vi "Final.vi"() -> ()   [LabVIEW 2019]
doc: "The myRIO Project template acquires acceleration data from the onboard accelerometer and displays the changes of acceleration values in a waveform chart."
uses:
  <vilib>/myRIO/Instrument Drivers/Onboard IO/I2C/typedefs/I2C User Configuration.ctl
  <vilib>/myRIO/Instrument Drivers/Onboard IO/I2C/typedefs/I2C Transfer Rate.ctl
  <vilib>/Platform/TimedLoop/XDataNode/timing_clust.ctl
  <vilib>/Platform/TimedLoop/XDataNode/nitl_modes.ctl
  <vilib>/Platform/TimedLoop/XDataNode/wakeup.ctl
  <vilib>/myRIO/Instrument Drivers/Onboard Devices/Accelerometer/typedefs/Accelerometer Reference.ctl
  <vilib>/myRIO/Common/Instrument Driver Framework/Utilities/typedefs/myRIO Generic Hardware Reference.ctl
  <vilib>/myRIO/Common/Instrument Driver Framework/Utilities/typedefs/Hardware Version Enum.ctl
  <vilib>/myRIO/Common/Instrument Driver Framework/Utilities/typedefs/myRIO v1.0 Reference.ctl
  <vilib>/myRIO/Common/Instrument Driver Framework/Utilities/typedefs/Generic FPGA Reference.ctl
  <vilib>/myRIO/Common/Instrument Driver Framework/myRIO v1.0/Accelerometer/typedefs/Accelerometer Channels List.ctl
  <vilib>/myRIO/Common/Instrument Driver Framework/myRIO v1.0/Accelerometer/typedefs/Accelerometer Channels Enum.ctl
  <vilib>/userDefined/High Color/nirio_resource_hc.ctl
  <vilib>/myRIO/Instrument Drivers/Onboard IO/PWM/typedefs/PWM Reference.ctl
  <vilib>/myRIO/Common/Instrument Driver Framework/myRIO v1.0/PWM/typedefs/PWM Channels Enum.ctl
  <vilib>/myRIO/Instrument Drivers/Onboard IO/PWM/typedefs/PWM Configuration.ctl
  <vilib>/myRIO/Instrument Drivers/Onboard IO/DIO/typedefs/DIO Reference.ctl
  <vilib>/myRIO/Common/Instrument Driver Framework/myRIO v1.0/DIO/typedefs/DIO Channels List.ctl
  <vilib>/myRIO/Common/Instrument Driver Framework/myRIO v1.0/DIO/typedefs/DIO Channels Enum.ctl
  <vilib>/myRIO/Common/Instrument Driver Framework/Utilities/vis/Is FPGA Ref Available.vi
  <vilib>/myRIO/Common/Instrument Driver Framework/myRIO v1.0/Accelerometer/vis/myRIO v1.1 Open Accelerometer.vi
  <vilib>/myRIO/Common/Instrument Driver Framework/myRIO v1.0/PWM/vis/myRIO v1.1 Open PWM.vi
  <vilib>/myRIO/Instrument Drivers/Onboard IO/PWM/vis/Set Duty Cycle and Frequency.vi
  <vilib>/myRIO/Common/Instrument Driver Framework/myRIO v1.0/DIO/vis/myRIO v1.1 Open DIO.vi
  <vilib>/myRIO/Common/Instrument Driver Framework/myRIO v1.0/I2C/vis/myRIO v1.1 Open I2C.vi
  <vilib>/myRIO/Common/Instrument Driver Framework/Utilities/vis/Validate Channels.vi
  <vilib>/myRIO/Common/Instrument Driver Framework/myRIO v1.0/Accelerometer/vis/myRIO v1.0 Reserve Accelerometer.vi
  <vilib>/myRIO/Common/Instrument Driver Framework/myRIO v1.0/PWM/vis/myRIO v1.0 Reserve PWM.vi
  <vilib>/myRIO/Common/Instrument Driver Framework/myRIO v1.0/DIO/vis/myRIO v1.0 Reserve DIO.vi
  <vilib>/myRIO/Common/Instrument Driver Framework/myRIO v1.0/UART/vis/myRIO v1.0 Close UART.vi
  <vilib>/myRIO/Common/Instrument Driver Framework/myRIO v1.0/I2C/vis/myRIO v1.0 Reserve I2C.vi
  <vilib>/myRIO/Common/Instrument Driver Framework/myRIO v1.0/Resource Manager/vis/myRIO v1.0 Reserve Channel List.vi
  <vilib>/myRIO/Common/Instrument Driver Framework/myRIO v1.0/Accelerometer/vis/myRIO v1.0 Build MUX Configuration Accelerometer.vi
  <vilib>/myRIO/Common/Instrument Driver Framework/myRIO v1.0/PWM/vis/myRIO v1.0 Build MUX Configuration PWM.vi
  <vilib>/myRIO/Common/Instrument Driver Framework/myRIO v1.0/DIO/vis/myRIO v1.0 Build MUX Configuration DIO.vi
  <vilib>/myRIO/Common/Instrument Driver Framework/myRIO v1.0/I2C/vis/myRIO v1.0 Build MUX Configuration I2C.vi
  <vilib>/myRIO/Common/Instrument Driver Framework/myRIO v1.0/Resource Manager/vis/myRIO v1.0 Reserve Channel.vi
  <vilib>/myRIO/Common/Instrument Driver Framework/myRIO v1.0/Resource Manager/vis/myRIO v1.0 Unreserve Channel.vi
  <vilib>/myRIO/Common/Instrument Driver Framework/myRIO v1.0/Resource Manager/vis/myRIO v1.0 Create Configuration List.vi
  <vilib>/myRIO/Common/Instrument Driver Framework/myRIO v1.0/Resource Manager/vis/myRIO v1.0 Build Mutex Name.vi
  <vilib>/Utility/VariantDataType/GetNumericInfo.vi
  <vilib>/Utility/error.llb/Error Cluster From Error Code.vi
  <vilib>/myRIO/Common/Instrument Driver Framework/myRIO v1.0/myRIO v1.1 Open.vi
  <vilib>/myRIO/Common/Instrument Driver Framework/Utilities/vis/IO Manager.vi
  <vilib>/myRIO/Common/Instrument Driver Framework/Utilities/vis/Configuration Manager.vi
  <vilib>/myRIO/Common/Instrument Driver Framework/myRIO v1.0/Resource Manager/vis/myRIO v1.0 Configure IO.vi
  <vilib>/myRIO/Common/Instrument Driver Framework/myRIO v1.0/myRIO v1.0 Close.vi
  <vilib>/myRIO/Common/Instrument Driver Framework/myRIO v1.0/I2C/vis/myRIO v1.0 Configure I2C.vi
  <vilib>/myRIO/Common/Instrument Driver Framework/myRIO v1.0/I2C/vis/myRIO v1.0 Write I2C.vi
  <vilib>/myRIO/Common/Instrument Driver Framework/myRIO v1.0/Accelerometer/vis/myRIO v1.0 Get Scaling Constant Accelerometer.vi
  <vilib>/myRIO/Common/Instrument Driver Framework/myRIO v1.0/Accelerometer/vis/myRIO v1.0 Read Accelerometer.vi
  <vilib>/myRIO/Common/Instrument Driver Framework/myRIO v1.0/DIO/vis/myRIO v1.0 Read DIO.vi
  <vilib>/myRIO/Common/Instrument Driver Framework/myRIO v1.0/DIO/vis/myRIO v1.0 Write DIO.vi
  <vilib>/myRIO/Common/Instrument Driver Framework/myRIO v1.0/I2C/vis/myRIO v1.0 Read I2C.vi
  <vilib>/myRIO/Common/Instrument Driver Framework/myRIO v1.0/PWM/vis/myRIO v1.0 Write PWM.vi
  <vilib>/myRIO/Common/Instrument Driver Framework/Utilities/vis/FPGA Ref Manager.vi
  <vilib>/myRIO/Common/Instrument Driver Framework/myRIO v1.0/myRIO v1.0 Reset FPGA.vi
  <vilib>/myRIO/Common/Instrument Driver Framework/myRIO v1.0/IRQ/vis/myRIO v1.0 IRQ Info FGV.vi
  <vilib>/myRIO/Common/Instrument Driver Framework/myRIO v1.0/IRQ/vis/myRIO v1.0 Timer IRQ Info FGV.vi
  <vilib>/myRIO/Common/Instrument Driver Framework/myRIO v1.0/IRQ/vis/myRIO v1.0 ISR Agent.vi
  <vilib>/myRIO/Instrument Drivers/Utilities/vis/Reset Index.vi
  <vilib>/myRIO/Common/Instrument Driver Framework/myRIO v1.0/Resource Manager/vis/myRIO v1.0 Block Write Resource Manager.vi
  <vilib>/Platform/TimedLoop/XDataNode/XDataNode.xnode
  <vilib>/myRIO/Express VI/Onboard Devices/Accelerometer/Accelerometer Express VI.xnode
  <vilib>/myRIO/Instrument Drivers/Onboard Devices/Accelerometer/vis/myRIO Accelerometer Open.xnode
  <vilib>/myRIO/Express VI/Onboard IO/PWM/PWM Express VI.xnode
  <vilib>/myRIO/Instrument Drivers/Onboard IO/PWM/vis/myRIO PWM Open.xnode
  <vilib>/myRIO/Express VI/Onboard IO/DO/DO Express VI.xnode
  <vilib>/myRIO/Instrument Drivers/Onboard IO/DIO/vis/myRIO DIO Open.xnode
  <vilib>/myRIO/Instrument Drivers/Onboard IO/I2C/I2C.lvlib
  <vilib>/myRIO/Instrument Drivers/Onboard IO/DIO/DIO.lvlib
  <vilib>/myRIO/Instrument Drivers/Utilities/Utilities.lvlib
  <vilib>/myRIO/Instrument Drivers/Onboard IO/PWM/PWM.lvlib
  <vilib>/addons/control/pid/NI_PID_autopid.lvlib
  <vilib>/Platform/TimedLoop/XDataNode/XDNodeRunTimeDep.lvlib
  <vilib>/myRIO/Instrument Drivers/Onboard Devices/Accelerometer/Accelerometer.lvlib
panel:
  out "output":dbl(graph) caption="출력"
  in  "[ESC]":bool
  out "X rate":i16
  out "Y rate":i16
  out "Z rate":i16
  out "DATA":u8[](array[numeric]) format="%02x"
  out "Angular rate [LSB/sec]":cluster{i16, i16, i16}(graph)
  in  "break":bool
  in  "dead":dbl format="%#_13g"
  out "abs(x)":dbl
  out "x*y":dbl
  out "숫자형 컨트롤 2":dbl
  in  "setpoint 2":dbl caption="셋포인트" format="%.2f"
  out "웨이브폼 차트 2":dbl(graph)
  in  "PID gains 3":T1={"proportional gain (Kc)"=1.0, "integral time (Ti, min)"=0.01, "derivative time (Td, min)"=0.0} {"proportional gain (Kc)" step=1.0; "integral time (Ti, min)" step=1.0; "derivative time (Td, min)" step=1.0}
  out "PID gains out":T1={"proportional gain (Kc)"=1.0, "integral time (Ti, min)"=0.01, "derivative time (Td, min)"=0.0} caption="PID 게인 출력" {"derivative time (Td, min)" format="%.3f"; "integral time (Ti, min)" format="%.3f"; "proportional gain (Kc)" format="%.3f"}
  in  "autotune? (F)":bool caption="자동튜닝? (거짓)"
  in  "autotuning parameters":T2={"controller type"=1, "relay cycles"=3, "relay amplitude"=1.0, "control specification"=2, "PV noise level"=0.1} caption="자동튜닝 파라미터" {"PV noise level" format="%.2f"; "control specification" items=["보통", "빠르게", "느리게"]; "relay amplitude" format="%.2f"; "controller type" items=["PID", "PI", "P"]}
  out "tuning completed?":bool caption="튜닝 완료?"
  out "dt out (s)":dbl caption="dt 출력 (초)" format="%.3f"
  in  "reinitialize? (F)":bool caption="다시 초기화? (거짓)"
  out "숫자형 컨트롤":dbl
  # "Overview: The myRIO Project template acquires acceleration data from the onboard accelerometer and displays the changes of acceleration values in a waveform chart.\nInstructions:\n1. Check the myRIO target IP address in the project and make sure the target IP address is correct. \n2. Run this VI."
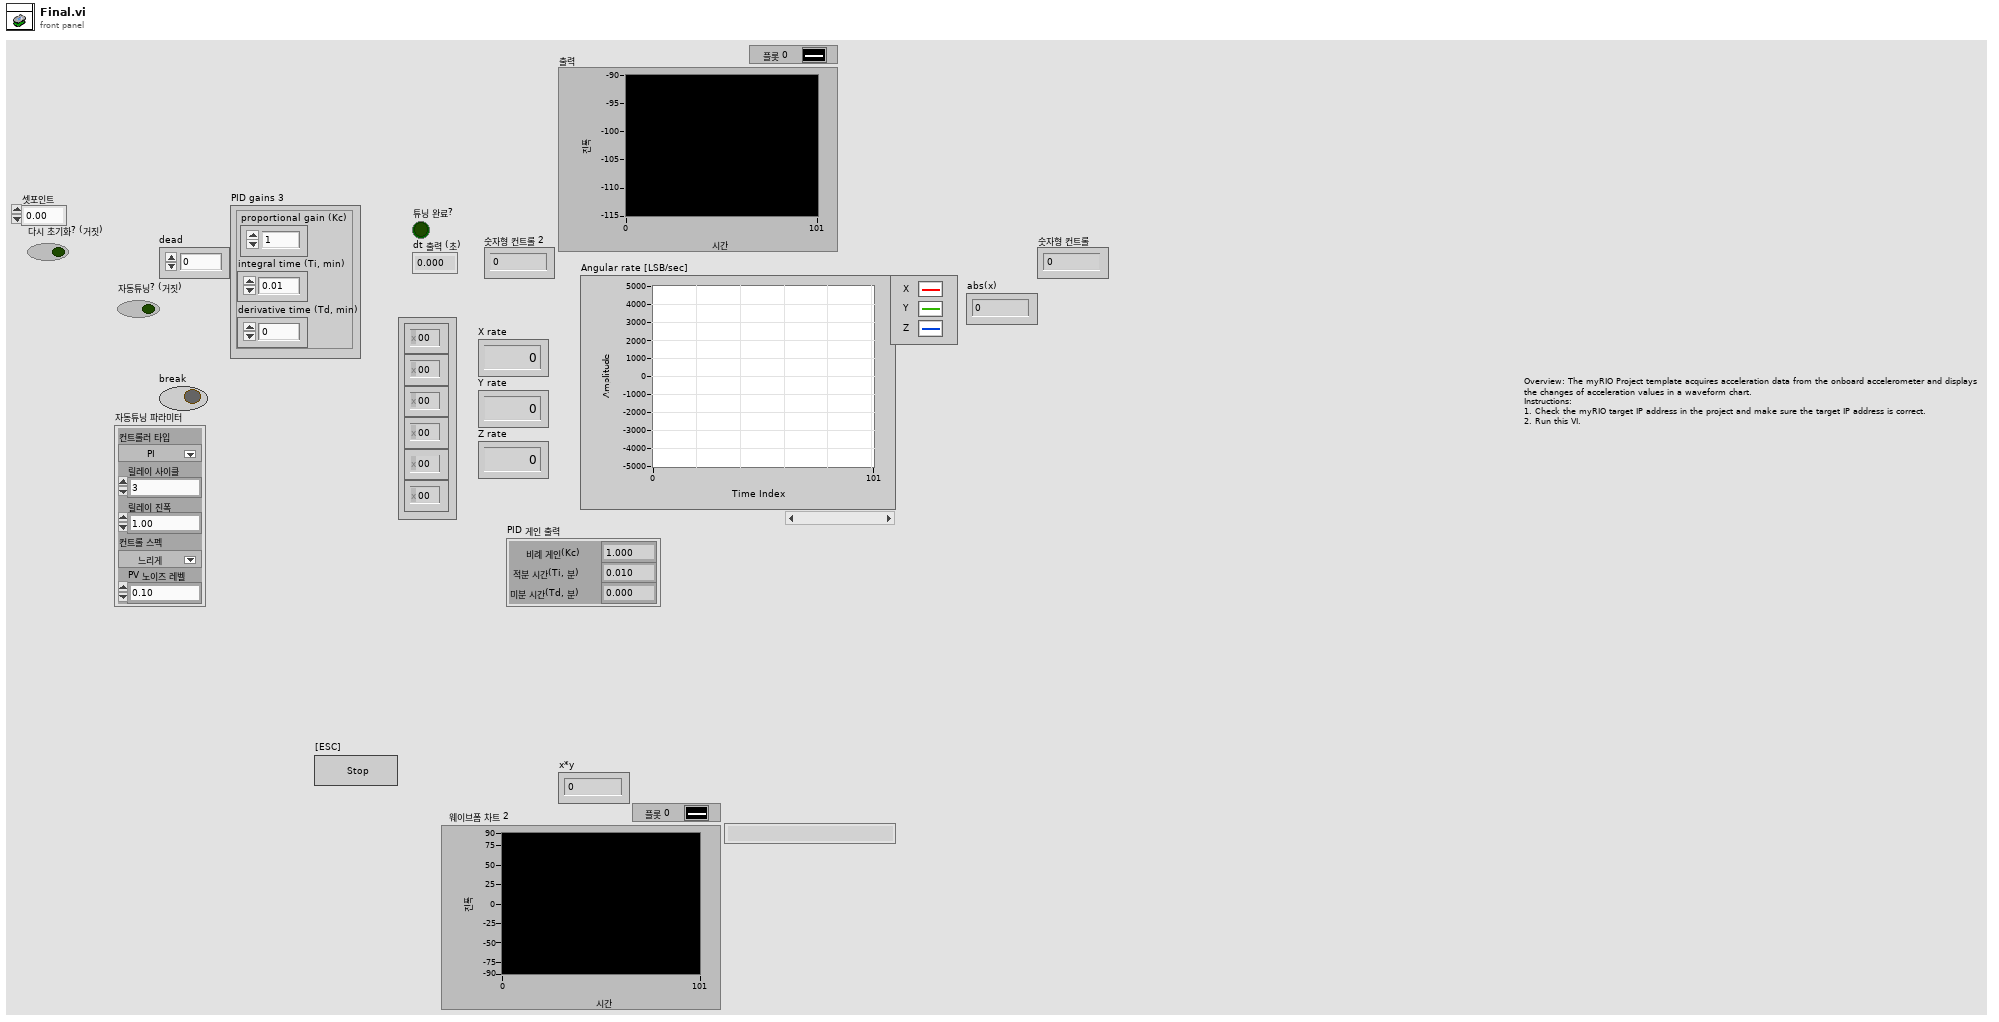
[diagram p1: front panel]
types:
  T1 = cluster{"proportional gain (Kc)":dbl, "integral time (Ti, min)":dbl, "derivative time (Td, min)":dbl}
  T2 = cluster{"controller type":u16, "relay cycles":i32, "relay amplitude":dbl, "control specification":u16, "PV noise level":dbl}
  T3 = typedef "I2C.lvlib/I2C User Configuration.ctl" = cluster{"I2C Transfer Rate":T4}
  T4 = typedef "I2C.lvlib/I2C Transfer Rate.ctl" = enum16{"Standard mode (100 kbps)", "Fast mode (400 kbps)"}
  T5 = typedef "I2C.lvlib/I2C Reference.ctl" = cluster{"myRIO Reference":T6, "I2C Channels Enum":T10, "I2C Configuration":T11}
  T6 = typedef "myRIO Generic Hardware Reference.ctl" = cluster{"myRIO Model":T7, "myRIO Hardware Reference":T8}
  T7 = typedef "Hardware Version Enum.ctl" = enum16{"Unknown", "myRIO-1900", "myRIO-1950", "roboRIO", "NI ELVIS RIO CM", "ELVIS III"}
  T8 = typedef "myRIO v1.0 Reference.ctl" = cluster{"Generic FPGA Reference":T9, "Allow multiple opens":bool}
  T9 = typedef "Generic FPGA Reference.ctl" = refnum<k20>
  T10 = typedef "I2C Channels Enum.ctl" = enum16{"Not Connected", "A/I2C", "B/I2C", "I2C/I2C"}
  T11 = typedef "I2C.lvlib/I2C Configuration.ctl" = cluster{"I2C Transfer Rate":T4}
  T12 = typedef "DIO.lvlib/DIO Reference.ctl" = cluster{"myRIO Reference":T6, "DIO Channels List":T13}
  T13 = typedef "DIO Channels List.ctl" = T14[]
  T14 = typedef "DIO Channels Enum.ctl" = enum16{"Not Connected", "C/DIO0", "C/DIO1", "C/DIO2", "C/DIO3", "C/DIO4", "C/DIO5", "C/DIO6", "C/DIO7", "A/DIO0", "A/DIO1", "A/DIO2", "A/DIO3", "A/DIO4", "A/DIO5", "A/DIO6", "A/DIO7", "A/DIO8", "A/DIO9", "A/DIO10", "A/DIO11", "A/DIO12", "A/DIO13", "A/DIO14", "A/DIO15", "A/DIO16", "A/DIO17", "A/DIO18", "A/DIO19", "B/DIO0", "B/DIO1", "B/DIO2", "B/DIO3", "B/DIO4", "B/DIO5", "B/DIO6", "B/DIO7", "B/DIO8", "B/DIO9", "B/DIO10", "B/DIO11", "B/DIO12", "B/DIO13", "B/DIO14", "B/DIO15", "B/DIO16", "B/DIO17", "B/DIO18", "B/DIO19", "LED0", "LED1", "LED2", "LED3", "Button0", "DIO/DIO0", "DIO/DIO1", "DIO/DIO2", "DIO/DIO3", "DIO/DIO4", "DIO/DIO5", "DIO/DIO6", "DIO/DIO7", "DIO/DIO8", "DIO/DIO9", "SPI/CS0", "SPI/CS1", "SPI/CS2", "SPI/CS3", "LED RADIO (Green)", "LED RADIO (Red)", "LED COMM (Green)", "LED COMM (Red)", "LED MODE (Green)", "LED MODE (Red)"}
  T15 = typedef "XDNodeRunTimeDep.lvlib/timing_clust.ctl" = cluster{"Expected End [f-1]":u64, "Actual End [f-1]":u64, "Finished Late? [f-1]":bool, "Expected End [i-1]":u64, "Actual End [i-1]":u64, "Finished Late? [i-1]":bool, "Expected Start [i]":u64, "Actual Start [i]":u64, "Expected Start [f]":u64, "Actual Start [f]":u64, "Source Name":string, "Structure Name":string, "Period":i64, "Deadline":i64, "Offset":i64, "Start":i64, "Priority":i32, "Timeout":i32, "Mode":T16, "Wakeup Reason":T17, "Error":errorcluster, "Source Type":string, "Secondary Source Type":string, "Global End Time":u64, "Global Start Time":u64, "Frame Duration":u64, "Iteration Duration":u64, "Assigned CPU":i32, "I/O Scan Engine Mode":u32}
  T16 = typedef "XDNodeRunTimeDep.lvlib/nitl_modes.ctl" = enum32{"No Change", "Process missed periods, maintain original phase", "Discard missed periods, maintain original phase", "Process missed periods, ignore original phase", "Discard missed periods, ignore original phase"}
  T17 = typedef "XDNodeRunTimeDep.lvlib/wakeup.ctl" = enum32{"Normal", "Aborted", "Asynchronous wakeup", "Timing source error", "Timed loop error", "Timeout"}
  T18 = typedef "Accelerometer.lvlib/Accelerometer Reference.ctl" = cluster{"myRIO Reference":T6, "Accelerometer Channels List":T19, "LSB Weight":dbl}
  T19 = typedef "Accelerometer Channels List.ctl" = T20[]
  T20 = typedef "Accelerometer Channels Enum.ctl" = enum16{"Not Connected", "X-Axis", "Y-Axis", "Z-Axis"}
  T21 = typedef "nirio_resource_hc.ctl" = tag
  T22 = typedef "PWM.lvlib/PWM Reference.ctl" = cluster{"myRIO Reference":T6, "PWM Channels Enum":T23, "PWM Configuration":T24}
  T23 = typedef "PWM Channels Enum.ctl" = enum16{"Not Connected", "C/PWM0", "C/PWM1", "A/PWM0", "A/PWM1", "A/PWM2", "A/PWM3", "A/PWM4", "A/PWM5", "A/PWM6", "A/PWM7", "A/PWM8", "A/PWM9", "A/PWM10", "A/PWM11", "A/PWM12", "A/PWM13", "A/PWM14", "A/PWM15", "A/PWM16", "A/PWM17", "A/PWM18", "A/PWM19", "B/PWM0", "B/PWM1", "B/PWM2", "B/PWM3", "B/PWM4", "B/PWM5", "B/PWM6", "B/PWM7", "B/PWM8", "B/PWM9", "B/PWM10", "B/PWM11", "B/PWM12", "B/PWM13", "B/PWM14", "B/PWM15", "B/PWM16", "B/PWM17", "B/PWM18", "B/PWM19", "PWM/PWM0", "PWM/PWM1", "PWM/PWM2", "PWM/PWM3", "PWM/PWM4", "PWM/PWM5", "PWM/PWM6", "PWM/PWM7", "PWM/PWM8", "PWM/PWM9"}
  T24 = typedef "PWM.lvlib/PWM Configuration.ctl" = cluster{"Frequency":dbl, "Duty Cycle":dbl}
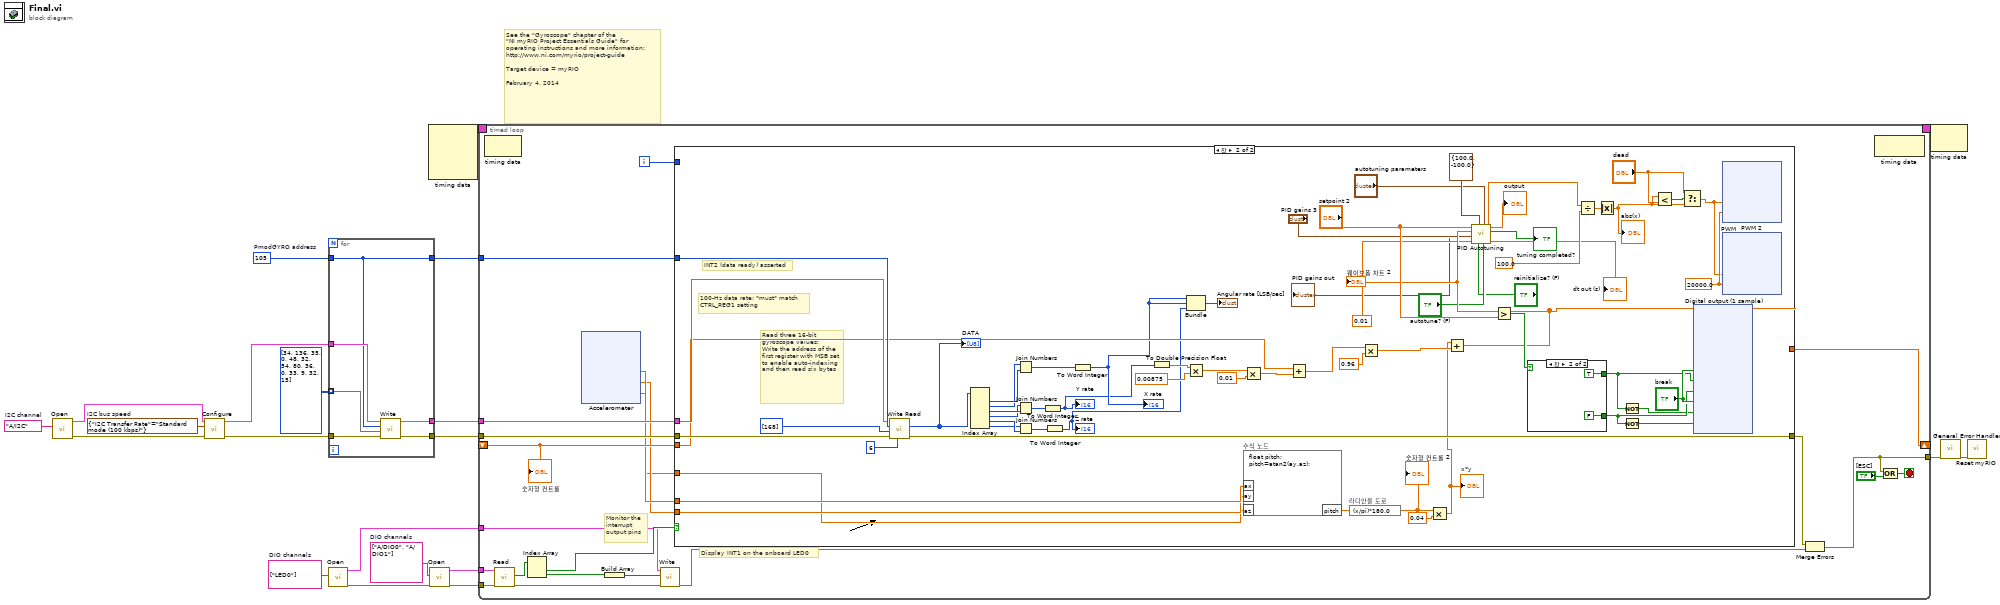
[diagram p0: block diagram]
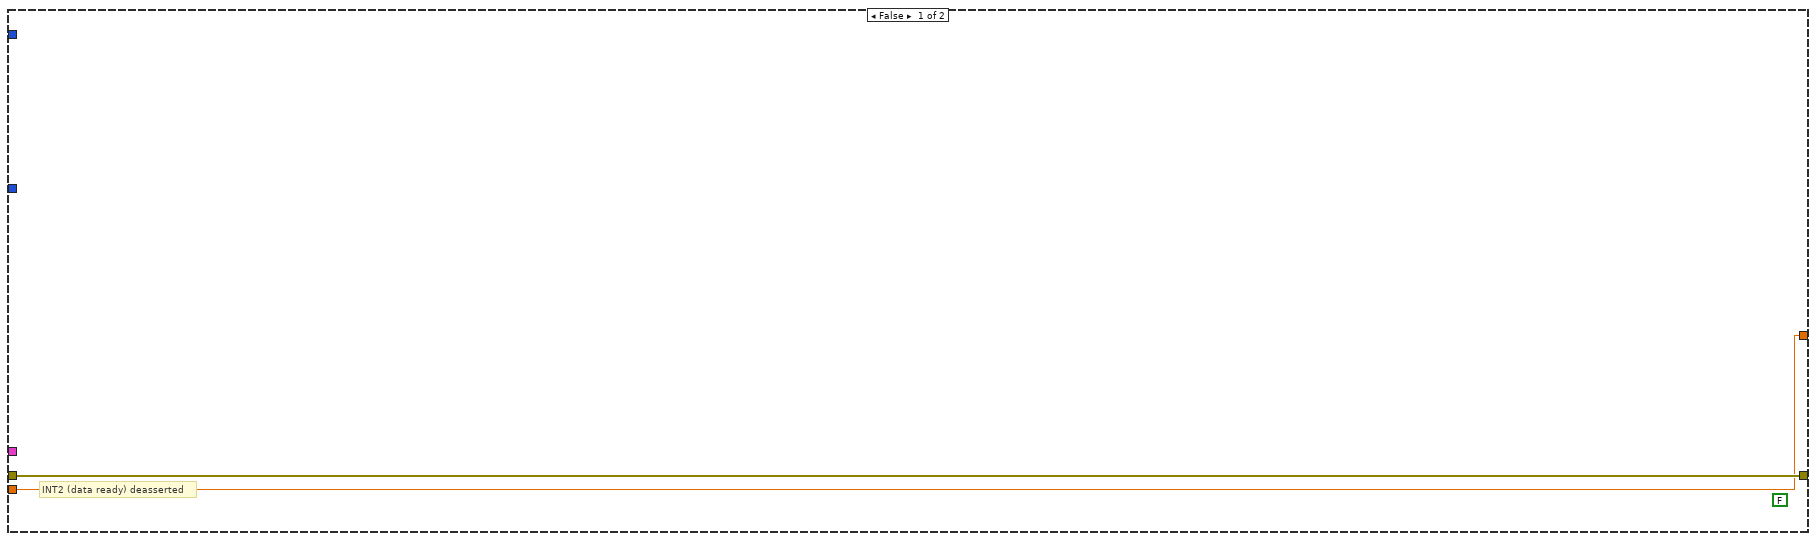
[diagram p2: hidden frame]
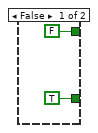
[diagram p3: hidden frame]
diagram:
  w5 = tag[] ["LED0"]  # DIO channels
  w6 = tag[] ["A/DIO0", "A/DIO1"]  # DIO channels
  w18 = T3 {"I2C Transfer Rate"=enum."Standard mode (100 kbps)"}  # I2C bus speed
  w19 = tag "A/I2C"  # I2C channel
  w9 = u8 105  # PmodGYRO address
  # "See the \"Gyroscope\" chapter of the\n\"NI myRIO Project Essentials Guide\" for\noperating instructions and more information: \nhttp://www.ni.com/myrio/project-guide\n\nTarget device = myRIO\n\nFebruary 4, 2014"
  n1 = call <vilib>:"Open.vi"("Channel Name"=w19) -> ("error out"=w16:errorcluster, "I2C Ref Out"=w17:T5)  [unwired: 9 in]
  n2 = call <vilib>:"Configure.vi"("error in (no error)"=w16, "I2C User Configuration"=w18, "I2C Ref In"=w17) -> ("error out"=w10:errorcluster, "I2C Ref Out"=w11:T5)  [unwired: 7 in]
  n3 = for {
    tunnel: [w27] -> w15
    tunnel: [w26] -> w14
    tunnel: [w22] -> w13
    tunnel: u8[][] [[34, 136], [35, 0], [48, 32], [54, 80], [36, 0], [33, 9], [32, 15]] ("Bytes to Write") -> [w25] mode=indexing
    tunnel: w11 -> [w24]
    tunnel: w10 -> [w23]
    tunnel: w9 -> [w22]
    n4 = call <vilib>:"Write.vi"("error in (no error)"=w23, "Bytes to Write"=w25, "Slave Address (7-bit)"=w22, "I2C Ref In"=w24) -> ("error out"=w27:errorcluster, "I2C Ref Out"=w26:T5)  [unwired: 6 in]
  }
  n5 = call <vilib>:"Open.vi"("Channel Names"=w5) -> ("error out"=w3:errorcluster, "DIO Ref Out"=w4:T12)  [unwired: 9 in]
  n6 = node-c288() -> (w21:T15)  [unwired: 4 in]
  n7 = call <vilib>:"Open.vi"("error in (no error)"=w3, "Channel Names"=w6) -> ("error out"=w8:errorcluster, "DIO Ref Out"=w7:T12)  [unwired: 8 in]
  n8 = timed-loop {
    tunnel: [w35] -> w1
    tunnel: w13 -> [w47]
    tunnel: w15 -> [w49]
    tunnel: w14 -> [w48]
    tunnel: w8 -> [w46]
    tunnel: w7 -> [w45]
    tunnel: w4 -> [w41]
    shift-right: [w37] -> _
    shift-left: _ -> [w36]
    timing: w21 -> [_]
    timing-out: [_] -> w20
    i -> [w31]
    stop <- w33 stop-if-true
    # "Display INT1 on the onboard LED0"
    # "Monitor the\ninterrupt\noutput pins"
    n9 = node-c288() -> ()  [unwired: 1 in, 1 out]
    n10 = call <vilib>:"Read.vi"("error in (no error)"=w46, "DIO Ref In"=w45) -> ("error out"=w40:errorcluster, "Values"=w42:bool[])  [unwired: 7 in, 1 out]
    n11 = Index Array "Index Array"(array=w42) -> (element #1=w43:bool, element #2=w38:bool)  [unwired: 2 in]
    n12 = xnode "Accelerometer"() -> ("X-Axis"=w30:dbl, "Y-Axis"=w29:dbl, "Z-Axis"=w28:dbl)  [unwired: 1 in, 1 out]
    n13 = Build Array "Build Array"(w38) -> (w39:bool[])
    n14 = call <vilib>:"Write.vi"("error in (no error)"=w40, "Values"=w39, "DIO Ref In"=w41) -> ("error out"=w32:errorcluster)  [unwired: 6 in, 1 out]
    n15 = case shown="참" w43 {
      tunnel: w49 -> [w92 w137]
      tunnel: w48 -> [_ w138]
      tunnel: w47 -> [_ w141]
      tunnel: [w92 w140] -> w44
      tunnel: [w91 w103] -> w37
      tunnel: w36 -> [w91 w130]
      tunnel: w31 -> [_ _]
      tunnel: w30 -> [_ w110]
      tunnel: w29 -> [_ w109]
      tunnel: w28 -> [_ w108]
      frame False {
        (unwired) FALSE
        # "INT2 (data ready) deasserted"
      }
      frame True {
        w117 = 20000.0 ("Frequency [Hz]")
        # "100-Hz data rate; *must* match\nCTRL_REG1 setting"
        # "INT2 (data ready) asserted"
        # "Read three 16-bit gyroscope values:\nWrite the address of the first register with MSB set to enable auto-indexing and then read six bytes"
        n16 = call <vilib>:"Write Read.vi"("Byte Count"=u32 6, "error in (no error)"=w137, "Bytes to Write"=u8[] [168], "Slave Address (7-bit)"=w141, "I2C Ref In"=w138) -> ("error out"=w140:errorcluster, "Bytes Read"=w139:u8[])  [unwired: 3 in, 1 out]
        "DATA" <- w139
        n17 = Index Array "Index Array"(array=w139) -> (element #1=w149:u8, element #2=w148:u8, element #3=w147:u8, element #4=w146:u8, element #5=w145:u8, element #6=w144:u8)  [unwired: 6 in]
        n18 = Join Numbers(hi=w148, lo=w149) -> ((hi.lo)=w153:u16)
        n19 = Join Numbers(hi=w146, lo=w147) -> ((hi.lo)=w152:u16)
        n20 = Join Numbers(hi=w144, lo=w145) -> ((hi.lo)=w151:u16)
        n21 = To Word Integer(number=w152) -> (16bit integer=w105:i16)
        "Y rate" <- w105
        n22 = To Word Integer(number=w151) -> (16bit integer=w111:i16)
        "Z rate" <- w111
        n23 = To Word Integer(number=w153) -> (16bit integer=w106:i16)
        "X rate" <- w106
        n24 = To Double Precision Float(number=w105) -> (double precision float=w113:dbl)
        n25 = Bundle "Bundle"(w106, w106, w111) -> (→"Angular rate [LSB/sec]":cluster{i16, i16, i16})  [unwired: 1 in]
        n26 = Multiply(x=w113, y=0.00875) -> (x*y=w126:dbl)
        n27 = formula code="float pitch;\npitch=atan2(ay,az);" "수식 노드"("ax"=w110, "az"=w108, "ay"=w109) -> ("pitch"=w132:dbl)
        n28 = Multiply(x=w126, y=0.01) -> (x*y=w127:dbl)
        n29 = Add(x=w130, y=w127) -> (x+y=w129:dbl)
        n30 = expression code="(x/pi)*180.0" "라디안을 도로"(w132) -> (w131:dbl)
        "숫자형 컨트롤 2" <- w131
        n31 = Multiply(x=w129, y=0.96) -> (x*y=w133:dbl)
        n32 = Multiply(x=w131, y=0.04) -> (x*y=w112:dbl)
        "x*y" <- w112
        n33 = Add(x=w112, y=w133) -> (x+y=w103:dbl)
        "웨이브폼 차트 2" <- w103
        n34 = call <vilib>:"PID Autotuning.vi"("autotune? (F)"="autotune? (F)", "autotuning parameters"="autotuning parameters", "reinitialize? (F)"="reinitialize? (F)", "output range"=cluster{"output high":dbl, "output low":dbl} {"output high"=100.0, "output low"=-100.0}, "dt (s)"=0.01, "PID gains"="PID gains 3", "process variable"=w103, "setpoint"="setpoint 2") -> ("dt out (s)"=→"dt out (s)":dbl, "PID gains out"=→"PID gains out":T1, "tuning completed?"=→"tuning completed?":bool, "output"=w99:dbl)
        "output" <- w99
        n35 = Greater?(x=w103, y="setpoint 2") -> (0:w122:bool)
        n36 = case shown="참" w122 {
          tunnel: [FALSE TRUE] -> w121
          tunnel: [TRUE FALSE] -> w120
          frame False {
          }
          frame True {
          }
        }
        n37 = Divide(x=w99, y=100.0) -> (x/y=w124:dbl)
        n38 = Absolute Value(x=w124) -> (abs(x)=w114:dbl)
        "abs(x)" <- w114
        n39 = Not(x=w121) -> (.not. x?=w119:bool)
        n40 = Not(x=w120) -> (.not. x?=w118:bool)
        n41 = Less?(x=w114, y="dead") -> (x < y?=w116:bool)
        n42 = Select(t="dead", s=w116, f=w114) -> (s? t:f=w107:dbl)
        n43 = xnode "Digital output (1 sample)"("En (A/DIO2 (Pin 15))"="break", "in1 (A/DIO3 (Pin 17))"=w121, "in2 (A/DIO4 (Pin 19))"=w120, "En2 (A/DIO5 (Pin 21))"="break", "in1_2 (A/DIO6 (Pin 23))"=w119, "in2_2 (A/DIO7 (Pin 25))"=w118) -> ()  [unwired: 1 in, 1 out]
        n44 = xnode "PWM 2"("Duty Cycle"=w107, "Frequency [Hz]"=w117) -> ()  [unwired: 1 in, 1 out]
        n45 = xnode "PWM"("Duty Cycle"=w107, "Frequency [Hz]"=w117) -> ()  [unwired: 1 in, 1 out]
      }
    }
    n46 = Merge Errors "Merge Errors"(w44, w32) -> (w35:errorcluster)
    n47 = node-c288() -> ()  [unwired: 1 in, 1 out]
    n48 = Compound Arithmetic op=OR ("복합 연산")(w35, "[ESC]") -> (w33:bool)
    "숫자형 컨트롤" <- w36
  }
  n49 = node-c288(w20) -> ()  [unwired: 1 out]
  n50 = call <vilib>:"General Error Handler.vi"("error in (no error)"=w1) -> ("error out"=w2:errorcluster)  [unwired: 10 in, 4 out]
  n51 = call <vilib>:"Reset myRIO.vi"("error in (no error)"=w2) -> ()  [unwired: 10 in, 1 out]
